vi "Task Init.vi"(8 "error in (no error)":errorcluster, 11 "VolatusCore in":refnum<class "VolatusCoreTask.lvclass">) -> (0 "error out":errorcluster, 3 "VolatusCore out":refnum<class "VolatusCoreTask.lvclass">)   [LabVIEW 2020, in "Volatus.lvlib" / "VolatusCoreTask.lvclass"]
uses:
  VolatusCoreTask.lvclass
  C:/Program Files (x86)/National Instruments/LabVIEW 2020/vi.lib/ActorFramework/Actor/Actor.lvclass
  C:/dev/lv20CE/relink/lv-volatus/Volatus/Task/Task.lvclass
  <vilib>/ActorFramework/Actor/Actor.lvclass/Actor.ctl
  <vilib>/ActorFramework/Message Enqueuer/Message Enqueuer.lvclass/Message Enqueuer.ctl
  VolatusCoreTask.lvclass/VolatusCoreTask.ctl
  <vilib>/ActorFramework/Message Enqueuer/Init from Existing Queue.vi
  VolatusAPI/VolatusAPI.lvclass
  C:/dev/lv20CE/relink/lv-volatus/Volatus/API/API.lvclass
  Task/Set Core APIs.vi
  <vilib>/ActorFramework/Message Enqueuer/Message Enqueuer.lvclass
  <vilib>/ActorFramework/Actor/Actor.lvclass
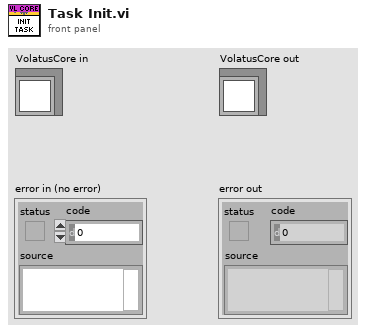
[diagram p1: front panel]
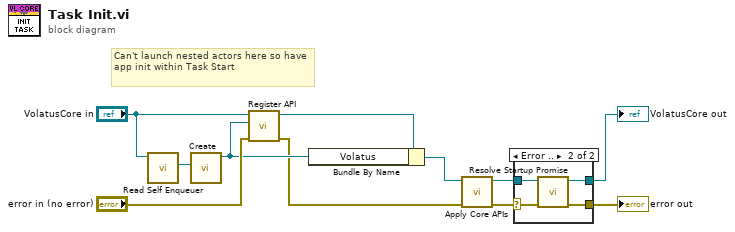
[diagram p0: block diagram]
diagram:
  # "Can't launch nested actors here so have app init within Task Start"
  n1 = call <vilib>:"Read Self Enqueuer.vi"("Actor"="VolatusCore in") -> ("Self Enqueuer"=w11:refnum<class "Message Enqueuer.lvclass">)  [unwired: 10 in]
  n2 = call "Create.vi"("EnQr"=w11) -> ("VolatusAPI out"=w7:refnum<class "VolatusAPI.lvclass">)  [unwired: 9 in, 1 out]
  n3 = call-dynamic "Register API.vi"("error in (no error)"="error in (no error)", "API"=w7, "VolatusCore in"="VolatusCore in") -> ("error out"=w2:errorcluster, "VolatusCore out"=w9:refnum<class "VolatusCoreTask.lvclass">)  [unwired: 7 in]
  n4 = Bundle By Name(cluster=w9, "Volatus"=w7) -> (w4:refnum<class "VolatusCoreTask.lvclass">)
  n5 = call "Apply Core APIs.vi"("error in (no error)"=w2, "VolatusCoreTask in"=w4) -> ("error out"=w1:errorcluster, "VolatusCoreTask out"=w3:refnum<class "VolatusCoreTask.lvclass">)  [unwired: 8 in]
  n6 = case shown="Error .." w1 {
    selector: w1 -> [w13 w17]
    tunnel: [w13 w16] -> w6
    tunnel: [w12 w15] -> w5
    tunnel: w3 -> [w12 w14]
    frame No Error {
    }
    frame Error {
      n7 = call "Resolve Startup Promise.vi"("error in (no error)"=w17, "VolatusCoreTask in"=w14) -> ("error out"=w16:errorcluster, "VolatusCoreTask out"=w15:refnum<class "VolatusCoreTask.lvclass">)  [unwired: 8 in]
    }
  }
  "error out" <- w6
  "VolatusCore out" <- w5
